vi "PhotonPipelineResult_PopulatePacket.vi"(11 "PhotonPipelineResult":T1 {"Targets"."CameraToTarget"."ROTATION"."SIN" format="%13.4f"; "Targets"."CameraToTarget"."ROTATION"."COS" format="%13.4f"; "Targets"."CameraToTarget"."ROTATION"."VALUE" format="%13.4f"; "Targets"."CameraToTarget"."TRANSLATION"."Y" format="%14.3f"; "Targets"."CameraToTarget"."TRANSLATION"."X" format="%14.3f"}) -> (3 "Packet_RawData":u8[](array[numeric]))   [LabVIEW 2019, in "PhotonVisionLib.lvlib"]
doc: "Convert a PipelineResult to a Packet array of bytes ready for writing to a Network Table variable.\n\nInputs:\n - PipelineResult -- PipelineResult cluster.\n\nOutputs:\n - Pacet_RawData -- Byte array containing the encoded PipelineResult."
uses:
  PhotonVisionLib.lvlib
  TypeDef/TargetCornerType.ctl
  TypeDef/PhotonTrackedTargetType.ctl
  TypeDef/PhotonPipelineResultType.ctl
  <vilib>/Rock Robotics/WPI/ThirdParty/JAS_Junk/TrajLib/TRANSLATION2D.ctl
  <vilib>/Rock Robotics/WPI/ThirdParty/JAS_Junk/TrajLib/Trajectory_Library.lvlib
  <vilib>/Rock Robotics/WPI/ThirdParty/JAS_Junk/TrajLib/ROTATION2D.ctl
  <vilib>/Rock Robotics/WPI/ThirdParty/JAS_Junk/TrajLib/TRANSFORM2D.ctl
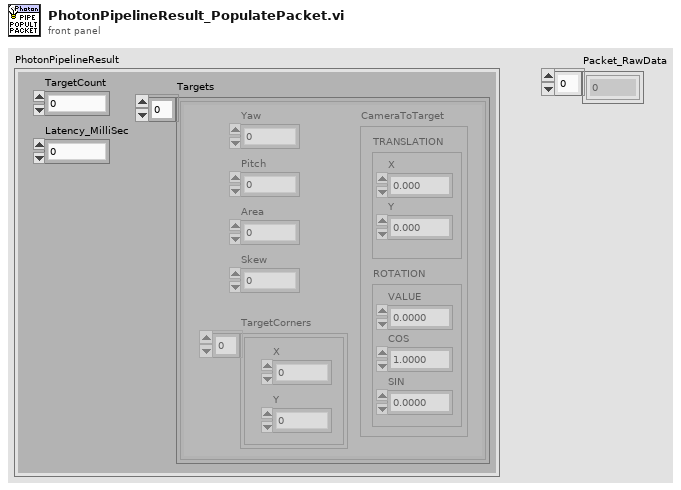
[diagram p1: front panel]
types:
  T1 = typedef "PhotonVisionLib.lvlib/PhotonPipelineResultType.ctl" = cluster{"TargetCount":i32, "Latency_MilliSec":dbl, "Targets":T2[]}
  T2 = typedef "PhotonVisionLib.lvlib/PhotonTrackedTargetType.ctl" = cluster{"Yaw":dbl, "Pitch":dbl, "Area":dbl, "Skew":dbl, "TargetCorners":T3[], "CameraToTarget":T4}
  T3 = typedef "PhotonVisionLib.lvlib/TargetCornerType.ctl" = cluster{"X":dbl, "Y":dbl}
  T4 = typedef "Trajectory_Library.lvlib/TRANSFORM2D.ctl" = cluster{"TRANSLATION":T5, "ROTATION":T6}
  T5 = typedef "Trajectory_Library.lvlib/TRANSLATION2D.ctl" = cluster{"X":dbl, "Y":dbl}
  T6 = typedef "Trajectory_Library.lvlib/ROTATION2D.ctl" = cluster{"VALUE":dbl, "COS":dbl, "SIN":dbl}
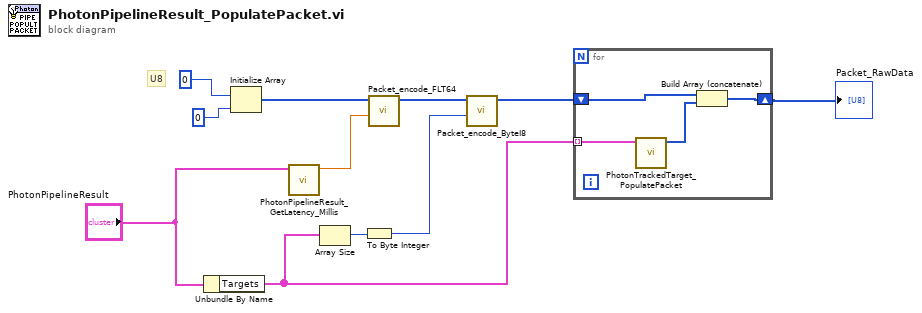
[diagram p0: block diagram]
diagram:
  # "U8"
  n1 = Unbundle By Name("PhotonPipelineResult") -> ("Targets"=w3:T2[])
  n2 = Initialize Array(u8 0 ("element"), 0 ("dimension size")) -> (w7:u8[])
  n3 = call "PhotonPipelineResult_GetLatency_Millis.vi"("PhotonPipelineResult"="PhotonPipelineResult") -> ("Latency_MilliSec"=w6:dbl)  [unwired: 10 in]
  n4 = Array Size(array=w3) -> (size(s)=w8:i32)
  n5 = To Byte Integer(number=w8) -> (8bit integer=w4:i8)
  n6 = call "Packet_encode_FLT64.vi"("FLT64_Value"=w6, "RawData In"=w7) -> ("RawData Out"=w5:u8[])  [unwired: 9 in]
  n7 = call "Packet_encode_ByteI8.vi"("Int8_Value"=w4, "RawData In"=w5) -> ("RawData Out"=w2:u8[])  [unwired: 9 in]
  n8 = for {
    tunnel: w3 -> [w15] mode=indexing
    shift-right: [w12] -> w1
    shift-left: w2 -> [w14]
    n9 = call "PhotonTrackedTarget_PopulatePacket.vi"("TrackedTarget"=w15) -> ("RawData Out"=w13:u8[])  [unwired: 10 in]
    n10 = Build Array (concatenate)(w14, w13) -> (w12:u8[])
  }
  "Packet_RawData" <- w1
